vi "RichToFlatnixnet_grpc_GetSubPropertyResponse.vi"(5 "OutputClusterType":T1, 11 "InputCluster":T2) -> (3 "OutputCluster":T1)   [LabVIEW 2025, in "grpc-xnet_client.lvlib"]
uses:
  nixnet_grpc_GetSubPropertyResponse.ctl
  nixnet_grpc_GetSubPropertyResponse_property_value/nixnet_grpc_GetSubPropertyResponse_property_value.lvclass
  nixnet_grpc_GetSubPropertyResponse_Flat.ctl
  grpc-xnet_client.lvlib
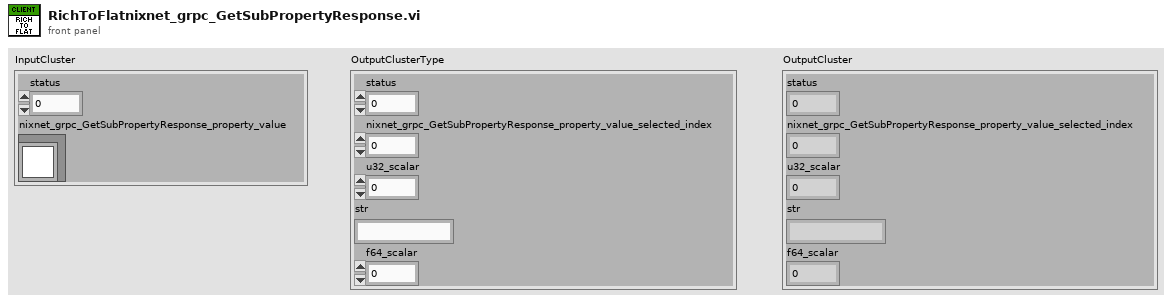
[diagram p1: front panel]
types:
  T1 = typedef "grpc-xnet_client.lvlib/nixnet_grpc_GetSubPropertyResponse_Flat.ctl" = cluster{"status":i32, "nixnet_grpc_GetSubPropertyResponse_property_value_selected_index":i32, "u32_scalar":u32, "str":string, "f64_scalar":dbl}
  T2 = typedef "grpc-xnet_client.lvlib/nixnet_grpc_GetSubPropertyResponse.ctl" = cluster{"status":i32, "nixnet_grpc_GetSubPropertyResponse_property_value":refnum<class "nixnet_grpc_GetSubPropertyResponse_property_value.lvclass">}
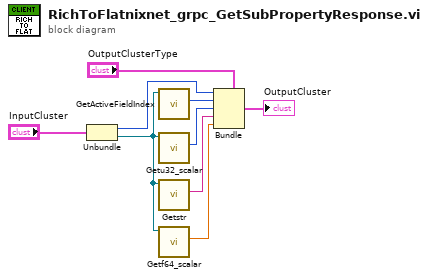
[diagram p0: block diagram]
diagram:
  n1 = Unbundle "Unbundle"("InputCluster") -> ("status"=w6:i32, "nixnet_grpc_GetSubPropertyResponse_property_value"=w5:refnum<class "nixnet_grpc_GetSubPropertyResponse_property_value.lvclass">)
  n2 = call "GetActiveFieldIndex.vi"("OneOfTemplate in"=w5) -> ("Active Field Index"=w4:i32)  [unwired: 8 in, 2 out]
  n3 = call "Getu32_scalar.vi"("OneOfTemplate in"=w5) -> ("Get_Val"=w3:u32)  [unwired: 8 in, 2 out]
  n4 = call "Getstr.vi"("OneOfTemplate in"=w5) -> ("Get_Val"=w2:string)  [unwired: 8 in, 2 out]
  n5 = call "Getf64_scalar.vi"("OneOfTemplate in"=w5) -> ("Get_Val"=w1:dbl)  [unwired: 8 in, 2 out]
  n6 = Bundle "Bundle"(cluster="OutputClusterType", "status"=w6, "nixnet_grpc_GetSubPropertyResponse_property_value_selected_index"=w4, "u32_scalar"=w3, "str"=w2, "f64_scalar"=w1) -> (→"OutputCluster":T1)
